vi "Get TestSuite Test Paths__core.vi"(8 "error in (no error)":errorcluster, 11 "Test Project":path) -> (0 "error out":errorcluster, 2 "Test Paths":path[](array[path]))   [LabVIEW 2011, in "GraphicalTestRunner.lvlib"]
uses:
  GraphicalTestRunner.lvlib
  Classes/TestLoader/TestLoader.lvclass
  Classes/TestSuite/TestSuite.lvclass
  <userlib>/_OpenG.lib/array/array.llb/Remove Duplicates from 1D Array (Path)__ogtk.vi
  JKI Reuse/Is an Error (error cluster)__jki_lib_error_handling -- VI Tester.vi
  Libraries/VITesterUtilities.lvlib
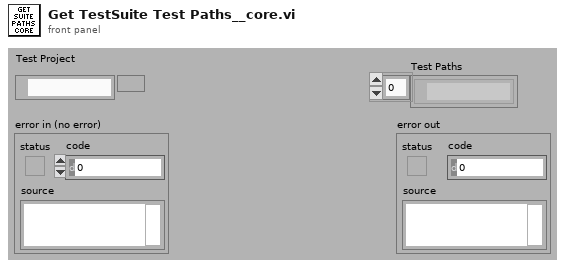
[diagram p1: front panel]
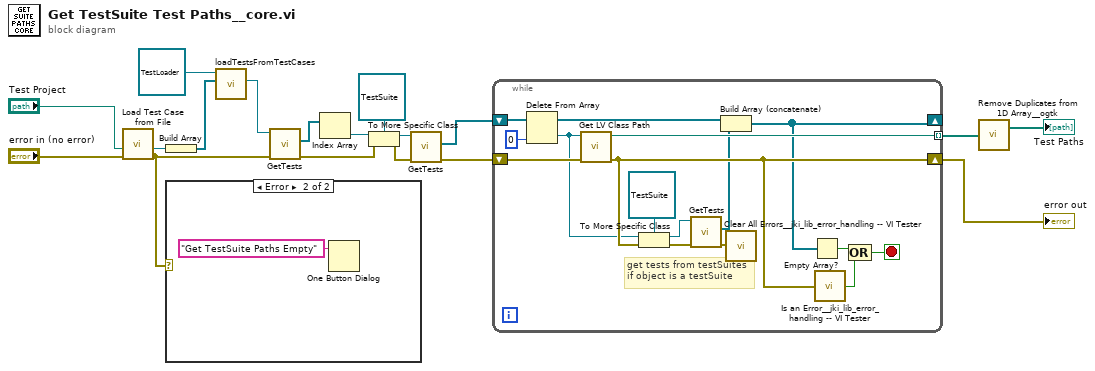
[diagram p0: block diagram]
diagram:
  n1 = call "Load Test Case from File.vi"("error in"="error in (no error)", "Test Class Path"="Test Project") -> ("error out"=w1:errorcluster, "Test"=w3:refnum<class>)  [unwired: 8 in]
  n2 = Build Array(w3) -> (w4:refnum<class>[])
  n3 = case shown="Error" w1 {
    frame No Error {
    }
    frame Error {
      n4 = One Button Dialog(message="Get TestSuite Paths Empty") -> ()  [unwired: 1 in, 1 out]
    }
  }
  n5 = call-dynamic "loadTestsFromTestCases.vi"("Tests"=w4, "TestLoader in"=refnum<class "TestLoader.lvclass"> refnum ("reference in")) -> ("TestSuite"=w5:refnum<class "TestSuite.lvclass">)  [unwired: 7 in, 2 out]
  n6 = call-dynamic "GetTests.vi"("error in (no error)"=w1, "TestSuite in"=w5) -> ("error out"=w11:errorcluster, "tests"=w6:refnum<class>[])  [unwired: 7 in, 1 out]
  n7 = Index Array(array=w6) -> (element=w7:refnum<class>)  [unwired: 1 in]
  n8 = To More Specific Class(target class=refnum<class "TestSuite.lvclass"> refnum ("TestSuite"), reference=w7, error in=w11) -> (specific class reference=w10:refnum<class "TestSuite.lvclass">, error out=w9:errorcluster)
  n9 = call-dynamic "GetTests.vi"("error in (no error)"=w9, "TestSuite in"=w10) -> ("error out"=w14:errorcluster, "tests"=w12:refnum<class>[])  [unwired: 7 in, 1 out]
  n10 = while {
    tunnel: [w35] -> w13 mode=indexing
    shift-right: [w24] -> w15
    shift-left: w14 -> [w34]
    shift-right: [w22] -> _
    shift-left: w12 -> [w33]
    stop <- w28 stop-if-true
    # "get tests from testSuites\nif object is a testSuite"
    n11 = Delete From Array(array=w33, index=0) -> (deleted portion=w23:refnum<class>, array with subset deleted=w31:refnum<class>[])  [unwired: 1 in]
    n12 = call <vilib>:"Get LV Class Path.vi"("error in (no error)"=w34, "object"=w23) -> ("error out"=w24:errorcluster, "class path"=w35:path)  [unwired: 8 in]
    n13 = To More Specific Class(target class=refnum<class "TestSuite.lvclass"> refnum ("TestSuite"), reference=w23, error in=w24) -> (specific class reference=w25:refnum<class "TestSuite.lvclass">, error out=w26:errorcluster)
    n14 = call-dynamic "GetTests.vi"("error in (no error)"=w26, "TestSuite in"=w25) -> ("error out"=w20:errorcluster, "tests"=w21:refnum<class>[])  [unwired: 7 in, 1 out]
    n15 = Build Array (concatenate)(w31, w21) -> (w22:refnum<class>[])
    n16 = call "Clear All Errors__jki_lib_error_handling -- VI Tester.vi"("error in"=w20) -> ()  [unwired: 4 in, 1 out]
    n17 = Empty Array?(array=w22) -> (empty?=w30:bool)
    n18 = call-poly "Is an Error__jki_lib_error_handling -- VI Tester.vi"("error in"=w24) -> ("error?"=w29:bool)  [unwired: 8 in]
    n19 = Compound Arithmetic op=OR(w30, w29) -> (w28:bool)
  }
  "error out" <- w15
  n20 = call-poly <userlib>:"Remove Duplicates from 1D Array__ogtk.vi"("Input Array"=w13) -> ("Output Array"=→"Test Paths":path[])  [unwired: 1 out]
